vi "Destroy.vi"(0 "reference in":refnum<class "AdvSigProc.lvclass">, 5 "error in (no error)":errorcluster) -> (14 "reference out":refnum<class "AdvSigProc.lvclass">, 19 "error out":errorcluster)   [LabVIEW 2020, in "AdvSigProc.lvclass"]
doc: "Destructor."
uses:
  AdvSigProc.lvclass
  API/Generic Utilities_class/Generic Utilities.lvclass
  API/GSwFormDSP_class/GSwFormDSP.lvclass
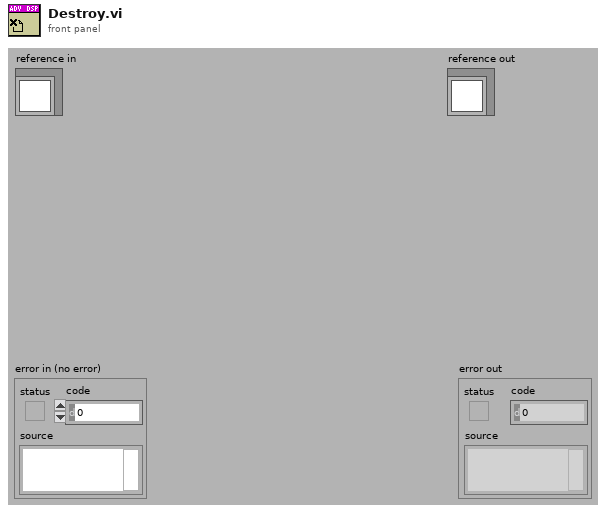
[diagram p1: front panel]
types:
  T1 = typedef "AdvSigProc.lvclass/ObjectAttributes.ctl" = cluster{"Time Data":cluster{"New Time Data Obj?":bool, "GSwFormDSP":refnum<class "GSwFormDSP.lvclass">}, "LMS Parameters":T2}
  T2 = typedef "AdvSigProc.lvclass/LMS.ctl" = cluster{"adaptive filter Ref":refnum<k20>, "Filtered Signals":refnum<class "GSwFormDSP.lvclass">, "Filter Coefs":dbl[], "Input Parameters":T3, "Iteration Metrics":T4[]}
  T3 = typedef "AdvSigProc.lvclass/LMS Input Parameters.ctl" = cluster{"Type":enum16{"Normalized LMS", "LMS", "FIR Sign LMS", "FIR Fast Block LMS", "RLS", "QR - RLS"}, "Filter Class":enum16{"Noise Cancelling (BGN Ref)", "Noise Cancelling (Speech Ref)"}, "Filter Length":i32, "µ Parameters":cluster{"Type":enum16{"User Input", "Auto µ"}, "step size":dbl}, "Iterations":cluster{"Current":i32, "Maximum":i32}}
  T4 = typedef "AdvSigProc.lvclass/Iteration Metrics.ctl" = cluster{"Name":string, "Max":dbl, "Min":dbl, "Values History":dbl[]}
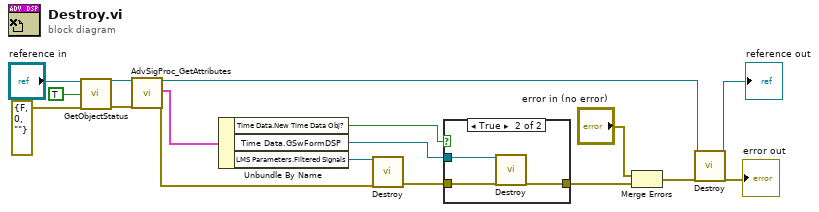
[diagram p0: block diagram]
diagram:
  n1 = call-dynamic "GetObjectStatus.vi"("reference in"="reference in", "simple info (F)"=TRUE ("simple info"), "error in (no error)"=errorcluster {"status"=FALSE, "code"=0, "source"=""}) -> ("reference out"=w11:refnum<class "AdvSigProc.lvclass">, "error out"=w12:errorcluster)  [unwired: 5 in, 10 out]
  n2 = call "AdvSigProc_GetAttributes.vi"("reference in"=w11, "error in (no error)"=w12) -> ("reference out"=w10:refnum<class "AdvSigProc.lvclass">, "attributes"=w5:T1, "error out"=w2:errorcluster)  [unwired: 14 in, 1 out]
  n3 = Unbundle By Name(w5) -> ("Time Data.New Time Data Obj?"=w6:bool, "Time Data.GSwFormDSP"=w7:refnum<class "GSwFormDSP.lvclass">, "LMS Parameters.Filtered Signals"=w3:refnum<class "GSwFormDSP.lvclass">)
  n4 = call-dynamic "Destroy.vi"("reference in"=w3, "error in (no error)"=w2) -> ("error out"=w1:errorcluster)  [unwired: 16 in, 1 out]
  n5 = case shown="True" w6 {
    tunnel: w7 -> [_ w21]
    tunnel: w1 -> [w18 w20]
    tunnel: [w18 w19] -> w4
    frame False {
    }
    frame True {
      n6 = call-dynamic "Destroy.vi"("reference in"=w21, "error in (no error)"=w20) -> ("error out"=w19:errorcluster)  [unwired: 16 in, 1 out]
    }
  }
  n7 = Merge Errors("error in (no error)", w4) -> (w16:errorcluster)
  n8 = call-parent "Destroy.vi"("reference in"=w10, "error in (no error)"=w16) -> ("reference out"=→"reference out":refnum<class "AdvSigProc.lvclass">, "error out"=→"error out":errorcluster)  [unwired: 16 in]
